vi "DMD_Sequence_Alloc_LUT18Bit_plusflash_.vi"(6 "nOffset":i32, 7 "LUT incl. diff":i32[](array[numeric]), 8 "error in (no error)":errorcluster, 10 "SequenceId":u32, 11 "DeviceId":u32) -> (0 "error out":errorcluster, 2 "SequenceId Out":u32, 3 "DeviceId Out":u32)   [LabVIEW 2020]
uses:
  <vilib>/Utility/error.llb/Error Cluster From Error Code.vi
  <userlib>/alp4395/alp4395.dll
panel:
  out "ControlValue":i32
  out "ALP_FLUT_ENTRIES9":i32
  out "ALP_FLUT_MAXENTRIES9":i32
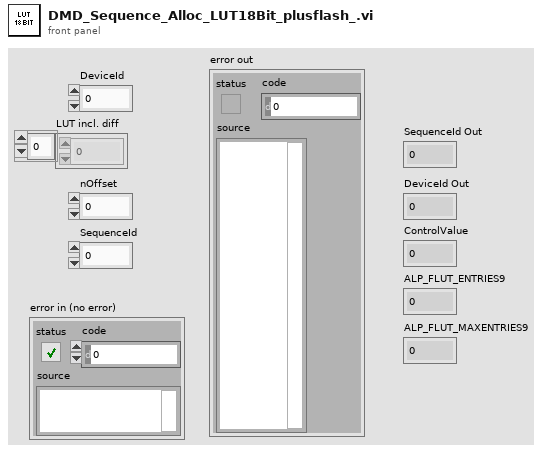
[diagram p1: front panel]
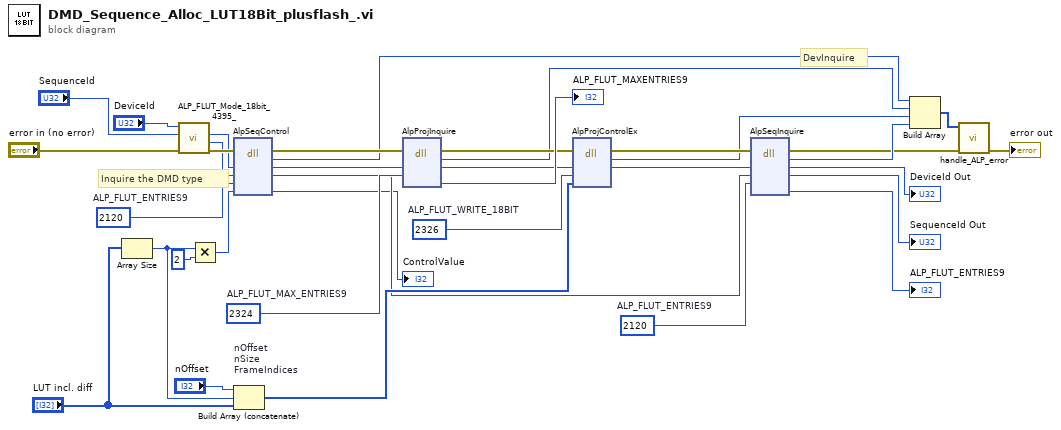
[diagram p0: block diagram]
diagram:
  w21 = 2120  # ALP_FLUT_ENTRIES9
  w11 = 2326  # ALP_FLUT_WRITE_18BIT
  w30 = 2120  # ALP_FLUT_ENTRIES9
  w33 = 2324  # ALP_FLUT_MAX_ENTRIES9
  # "DevInquire"
  # "Inquire the DMD type"
  n1 = Array Size(array="LUT incl. diff") -> (size(s)=w9:i32)
  n2 = call "ALP_FLUT_Mode_18bit_4395_.vi"("error in (no error)"="error in (no error)", "SequenceId in"="SequenceId", "DeviceId in"="DeviceId") -> ("error out"=w3:errorcluster, "SequenceId out"=w2:u32, "DeviceId out"=w1:u32)  [unwired: 6 in]
  n3 = Multiply(x=w9, y=2) -> (x*y=w8:i32)
  n4 = dll-call lib="C:/Program Files (x86)/National Instruments/LabVIEW 2020/user.lib/alp4395/alp4395.dll" fn="AlpSeqControl"(error in=w3, "DeviceId"=w1, "SequenceId"=w2, "ControlType"=w30, "ControlValue"=w8) -> (error out=w27:errorcluster, "return type"=w18:i32, "DeviceId"=w31:u32, "SequenceId"=w22:u32, "ControlValue"=→"ControlValue":i32)  [unwired: 3 in, 1 out]
  n5 = Build Array (concatenate) "nOffset\nnSize\nFrameIndices"("nOffset", w9, "LUT incl. diff") -> (w28:i32[])
  n6 = dll-call lib="C:/Program Files (x86)/National Instruments/LabVIEW 2020/user.lib/alp4395/alp4395.dll" fn="AlpProjInquire"(error in=w27, "DeviceId"=w31, "InquireType"=w33) -> (error out=w26:errorcluster, "return type"=w17:i32, "DeviceId"=w25:u32, "UserVar"=→"ALP_FLUT_MAXENTRIES9":i32)  [unwired: 4 in, 1 out]
  n7 = dll-call lib="C:/Program Files (x86)/National Instruments/LabVIEW 2020/user.lib/alp4395/alp4395.dll" fn="AlpProjControlEx"(error in=w26, "DeviceId"=w25, "ControlType"=w11, "UserStructPtr"=w28) -> (error out=w24:errorcluster, "return type"=w16:i32, "DeviceId"=w23:u32)  [unwired: 4 in, 1 out]
  n8 = dll-call lib="C:/Program Files (x86)/National Instruments/LabVIEW 2020/user.lib/alp4395/alp4395.dll" fn="AlpSeqInquire"(error in=w24, "DeviceId"=w23, "SequenceId"=w22, "InquireType"=w21) -> (error out=w14:errorcluster, "return type"=w15:i32, "DeviceId"=→"DeviceId Out":u32, "SequenceId"=→"SequenceId Out":u32, "UserVar"=→"ALP_FLUT_ENTRIES9":i32)  [unwired: 4 in, 1 out]
  n9 = Build Array(w18, w17, w16, w15) -> (w34:i32[])
  n10 = call "handle_ALP_error.vi"("error in"=w14, "Return Codes"=w34) -> ("error out"=→"error out":errorcluster)  [unwired: 9 in]
